vi "configure offset.vi"(7 "offset_val2":u32, 8 "error in (no error)":errorcluster, 9 "offset_val1":u32, 10 "Board":u16, 11 "identifier":string) -> (0 "error out":errorcluster, 2 "function return":u32, 3 "identifier out":string)   [LabVIEW 2015, in "XGL_DPP.lvlib"]
doc: "EXTERN DECLSPEC unsigned int CALL_CONV configure_offset(char* identifier, unsigned short Board, const configuration_offset const cfg_offset);"
uses:
  XGL_DPP.lvlib
  D:/Scanning Software_Demokritos_2015_v6/libs/XGL_DPP.dll
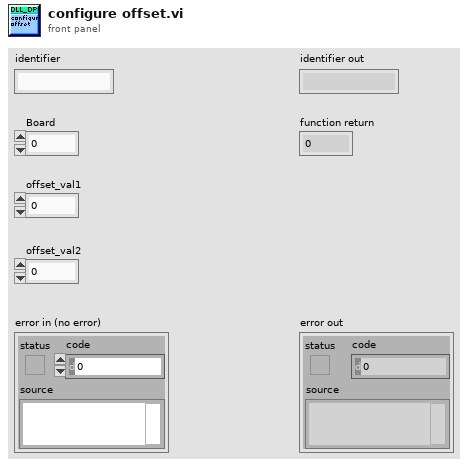
[diagram p1: front panel]
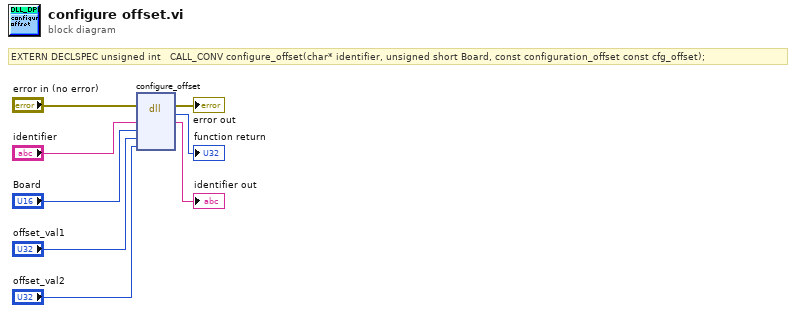
[diagram p0: block diagram]
diagram:
  # "EXTERN DECLSPEC unsigned int   CALL_CONV configure_offset(char* identifier, unsigned short Board, const configuration_offset const cfg_offset);"
  n1 = dll-call lib="D:/Scanning Software_Demokritos_2015_v6/libs/XGL_DPP.*" fn="configure_offset"(error in="error in (no error)", "identifier"="identifier", "Board"="Board", "offset_val1"="offset_val1", "offset_val2"="offset_val2") -> (error out=→"error out":errorcluster, "return type"=→"function return":u32, "identifier"=→"identifier out":string)  [unwired: 5 in, 1 out]
